vi "Day 06 (Part One).vi"() -> ()   [LabVIEW 2021]
panel:
  out "result":u32
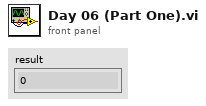
[diagram p1: front panel]
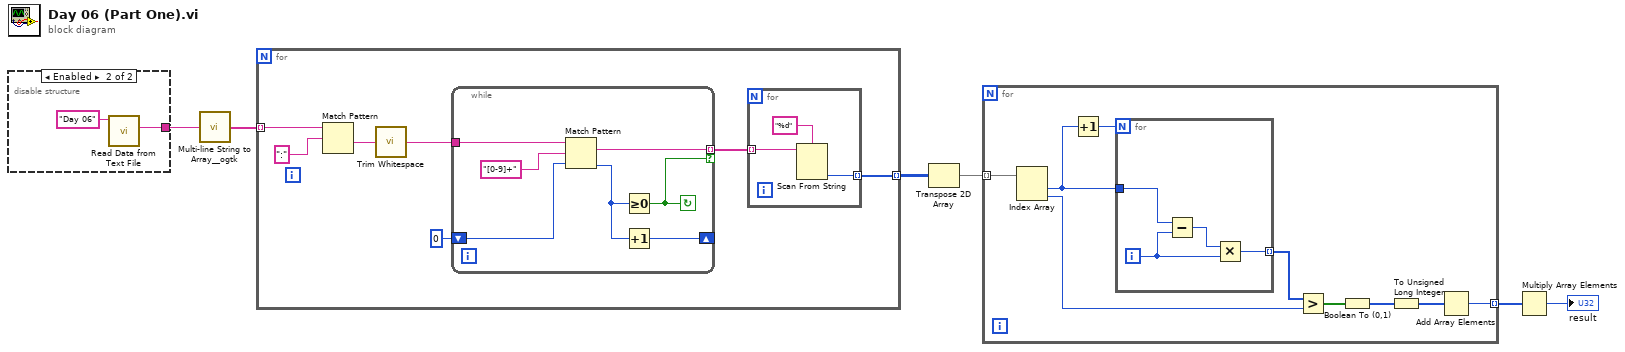
[diagram p0: block diagram]
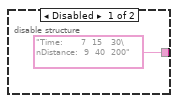
[diagram p2: hidden frame]
diagram:
  n1 = disable-structure shown="Enabled" {
    disable-tunnel: ["Time:      7  15   30\nDistance:  9  40  200" w9] -> w6
    frame Disabled {
    }
    frame Enabled {
      n2 = call "Read Data from Text File.vi"("Subfolder"="Day 06") -> ("data"=w9:string)  [unwired: 10 in]
    }
  }
  n3 = call <userlib>:"Multi-line String to Array__ogtk.vi"("string"=w6) -> ("lines"=w5:string[])
  n4 = for {
    tunnel: w5 -> [w16] mode=indexing
    tunnel: [w11] -> w4 mode=indexing
    n5 = Match Pattern(string=w16, regular expression=":") -> (after substring=w14:string)  [unwired: 1 in, 3 out]
    n6 = call <vilib>:"Trim Whitespace.vi"("string"=w14) -> ("trimmed string"=w13:string)  [unwired: 1 in]
    n7 = while {
      tunnel: w13 -> [w26]
      shift-right: [w24] -> _
      shift-left: 0 -> [w23]
      tunnel: [w20] -> w10 mode=indexing if=w21
      stop <- w21 continue-if-true
      n8 = Match Pattern(string=w26, regular expression="[0-9]+", offset (0)=w23) -> (match substring=w20:string, offset past match=w22:i32)  [unwired: 2 out]
      n9 = Greater Or Equal To 0?(x=w22) -> (x >= 0?=w21:bool)
      n10 = Increment(x=w22) -> (x+1=w24:i32)
    }
    n11 = for {
      tunnel: [w18] -> w11 mode=indexing
      tunnel: w10 -> [w17] mode=indexing
      n12 = Scan From String(format string="%d", input string=w17) -> (output 1=w18:i32)  [unwired: 3 in, 3 out]
    }
  }
  n13 = Transpose 2D Array(2D array=w4) -> (transposed array=w3:i32[][])
  n14 = for {
    tunnel: w3 -> [w35] mode=indexing
    tunnel: [w28] -> w2 mode=indexing
    n15 = Index Array(array=w35) -> (element #1=w33:i32, element #2=w31:i32)  [unwired: 2 in]
    n16 = Increment(x=w33) -> (x+1=w34:i32)
    n17 = for {
      N: w34 -> [_]
      tunnel: [w37] -> w32 mode=indexing
      tunnel: w33 -> [w36]
      i -> [w38]
      n18 = Subtract(x=w36, y=w38) -> (x-y=w39:i32)
      n19 = Multiply(x=w39, y=w38) -> (x*y=w37:i32)
    }
    n20 = Greater?(x=w32, y=w31) -> (0:w30:bool[])
    n21 = Boolean To (0,1)(Boolean=w30) -> (0, 1=w29:i16[])
    n22 = To Unsigned Long Integer(number=w29) -> (unsigned 32bit integer=w27:u32[])
    n23 = Add Array Elements(numeric array=w27) -> (sum=w28:u32)
  }
  n24 = Multiply Array Elements(1:w2) -> (0:→"result":u32)
